vi "Euclidean Norm.vi"(0 "X":dbl[](array[numeric]) format="%0.2f") -> (1 "root square value":dbl format="%0.2f", 2 "error":i32)   [LabVIEW 2020, in "NI_MAPro.lvlib"]
doc: "Finds the root-mean-square (RMS) of the input sequence X. The RMS value is computed using the following formula:\n\n RMS = sqrt( Sum{ X[i]^2 } / n).\n\n where \n n is the number of elements in X."
uses:
  NI_MAPro.lvlib
panel:
  # "Euclidian Norm"
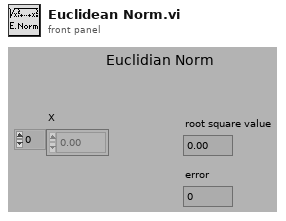
[diagram p1: front panel]
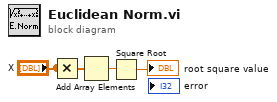
[diagram p0: block diagram]
diagram:
  n1 = Multiply(x="X", y="X") -> (x*y=w3:dbl[])
  n2 = Add Array Elements(numeric array=w3) -> (sum=w2:dbl)
  n3 = Square Root(x=w2) -> (sqrt(x)=→"root square value":dbl)
